vi "BuildStepListFromSteps.vi"(0 "Steps":T2(array[cluster]), 5 "Control Channels":string[](array[string]), 7 "Feedback Channels":string[](array[string]), 9 "AI":string[](array[string])) -> (4 "Step List":string[](array[string]))   [LabVIEW 2015]
panel:
  in  "Step":T1
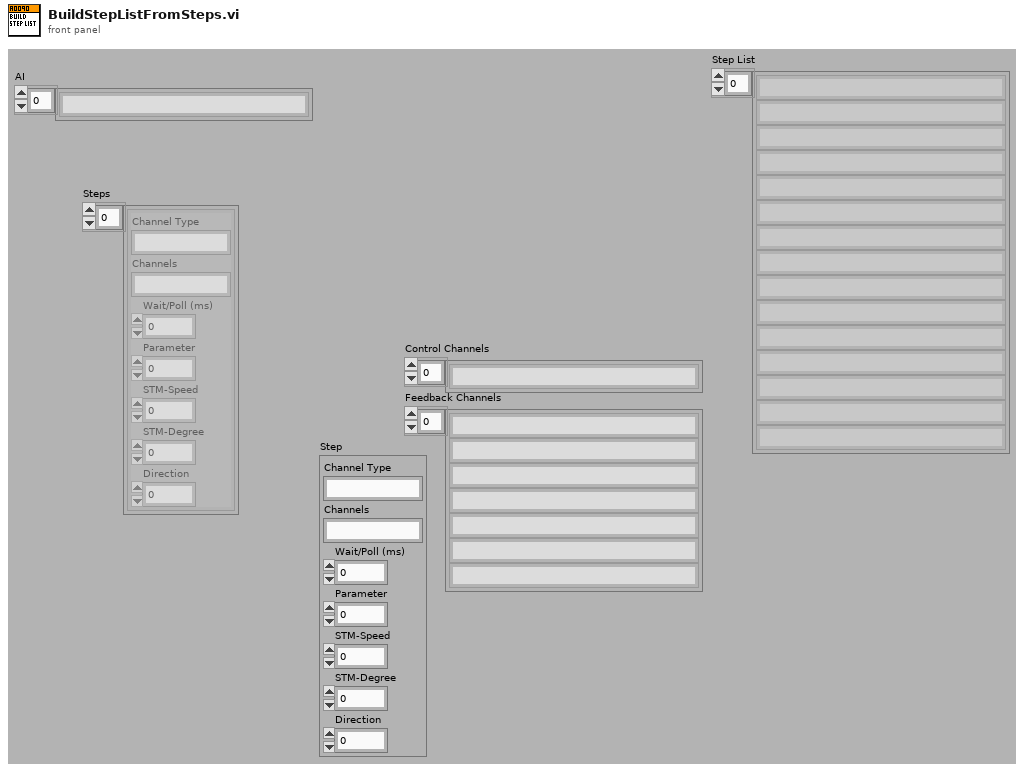
[diagram p1: front panel]
types:
  T1 = cluster{"Channel Type":string, "Channels":string, "Wait/Poll (ms)":u32, "Parameter":u8, "STM-Speed":u8, "STM-Degree":u32, "Direction":u8}
  T2 = cluster{"Channel Type":string, "Channels":string, "Wait/Poll (ms)":u32, "Parameter":u8, "STM-Speed":i32, "STM-Degree":u32, "Direction":u8}[]
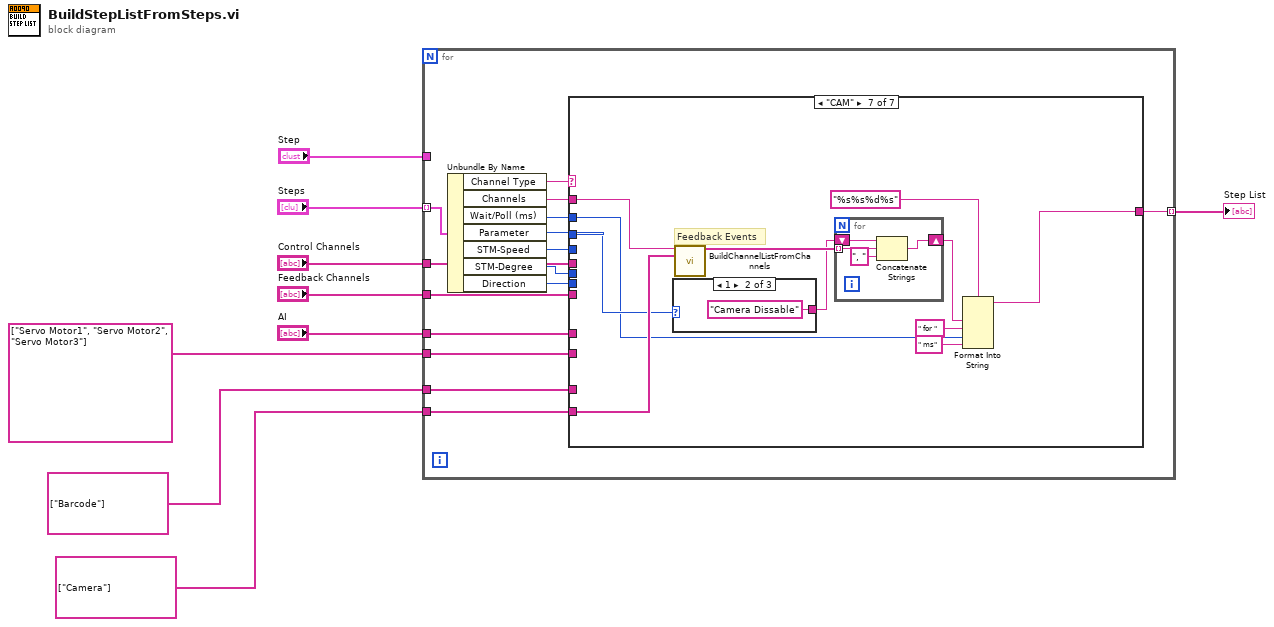
[diagram p0: block diagram]
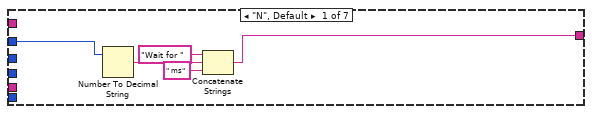
[diagram p2: hidden frame]
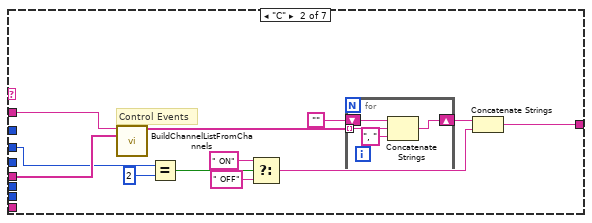
[diagram p3: hidden frame]
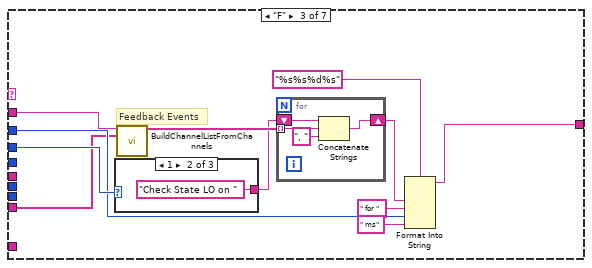
[diagram p4: hidden frame]
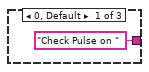
[diagram p5: hidden frame]
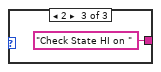
[diagram p6: hidden frame]
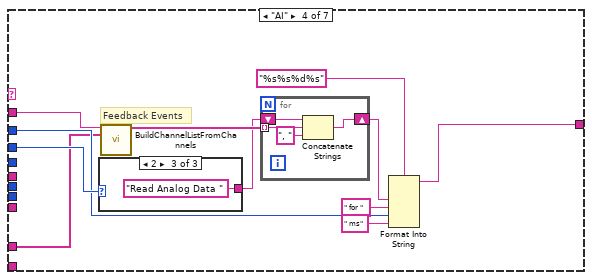
[diagram p7: hidden frame]
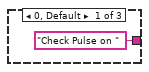
[diagram p8: hidden frame]
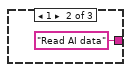
[diagram p9: hidden frame]
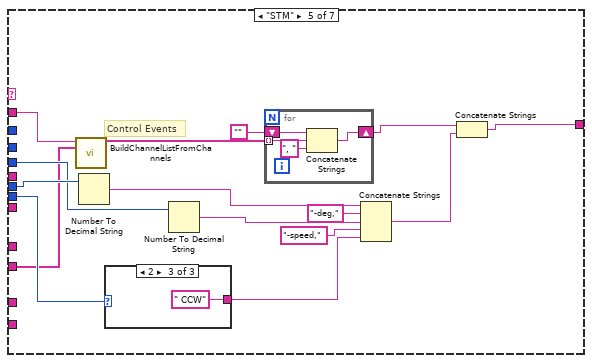
[diagram p10: hidden frame]
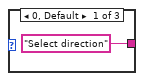
[diagram p11: hidden frame]
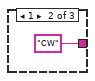
[diagram p12: hidden frame]
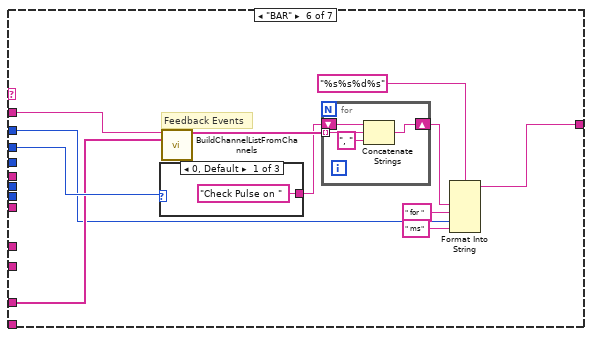
[diagram p13: hidden frame]
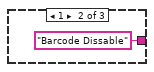
[diagram p14: hidden frame]
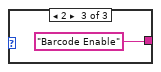
[diagram p15: hidden frame]
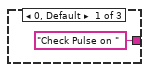
[diagram p16: hidden frame]
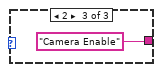
[diagram p17: hidden frame]
diagram:
  n1 = for {
    tunnel: "Steps" -> [w24] mode=indexing
    tunnel: "Control Channels" -> [w20]
    tunnel: "Feedback Channels" -> [w18]
    tunnel: [w17] -> w6 mode=indexing
    tunnel: "Step" -> [_]
    tunnel: "AI" -> [w16]
    tunnel: string[] ["Servo Motor1", "Servo Motor2", "Servo Motor3"] ("Control Channels 2") -> [w12]
    tunnel: string[] ["Barcode"] ("Channel Names (In)") -> [w11]
    tunnel: string[] ["Camera"] ("Channel Names (In)") -> [w10]
    n2 = Unbundle By Name(w24) -> ("Channel Type"=w23:string, "Channels"=w21:string, "Wait/Poll (ms)"=w22:u32, "Parameter"=w19:u8, "STM-Speed"=w13:i32, "STM-Degree"=w14:u32, "Direction"=w15:u8)
    n3 = case shown="\"CAM\"" w23 {
      tunnel: w22 -> [w26 _ w51 w67 _ w104 w123]
      tunnel: w21 -> [_ w41 w56 w66 w82 w107 w126]
      tunnel: w20 -> [_ w40 _ _ _ _ _]
      tunnel: w19 -> [_ w35 w52 w68 _ w108 w124]
      tunnel: w18 -> [_ _ w50 _ _ _ _]
      tunnel: [w25 w30 w47 w65 w92 w105 w122] -> w17
      tunnel: w16 -> [_ _ _ w64 _ _ _]
      tunnel: w15 -> [_ _ _ _ w93 _ _]
      tunnel: w14 -> [_ _ _ _ w91 _ _]
      tunnel: w13 -> [_ _ _ _ w88 _ _]
      tunnel: w12 -> [_ _ _ _ w83 _ _]
      tunnel: w11 -> [_ _ _ _ _ w106 _]
      tunnel: w10 -> [_ _ _ _ _ _ w125]
      frame "N", Default {
        n4 = Number To Decimal String(number=w26) -> (decimal integer string=w27:string)  [unwired: 1 in]
        n5 = Concatenate Strings("Wait for ", w27, " ms" ("string")) -> (w25:string)
      }
      frame "C" {
        # "Control Events"
        n6 = call "BuildChannelListFromChannels.vi"("Channels (A:B:C:D...) (In)"=w41, "Channel Names (In)"=w40) -> ("Channel List (Out)"=w34:string[])  [unwired: 12 in, 1 out]
        n7 = Equal?(x=w35, y=u8 2) -> (x = y?=w38:bool)
        n8 = Select(t=" ON", s=w38, f=" OFF") -> (s? t:f=w32:string)
        n9 = for {
          tunnel: w34 -> [w45] mode=indexing
          shift-right: [w42] -> w31
          shift-left: "" -> [w43]
          n10 = Concatenate Strings(w43, w45, ", " ("string")) -> (w42:string)
        }
        n11 = Concatenate Strings(w31, w32) -> (w30:string)
      }
      frame "F" {
        # "Feedback Events"
        n12 = case shown="1" w52 {
          tunnel: ["Check Pulse on " "Check State LO on " "Check State HI on "] -> w46
          frame 0, Default {
          }
          frame 1 {
          }
          frame 2 {
          }
        }
        n13 = call "BuildChannelListFromChannels.vi"("Channels (A:B:C:D...) (In)"=w56, "Channel Names (In)"=w50) -> ("Channel List (Out)"=w55:string[])  [unwired: 12 in, 1 out]
        n14 = for {
          tunnel: w55 -> [w63] mode=indexing
          shift-right: [w60] -> w48
          shift-left: w46 -> [w61]
          n15 = Concatenate Strings(w61, w63, ", " ("string")) -> (w60:string)
        }
        n16 = Format Into String(format string="%s%s%d%s", w48, " for " ("input 1"), w51, " ms" ("input 3")) -> (resulting string=w47:string)  [unwired: 2 in, 1 out]
      }
      frame "AI" {
        # "Feedback Events"
        n17 = case shown="2" w68 {
          tunnel: ["Check Pulse on " "Read AI data" "Read Analog Data "] -> w69
          frame 0, Default {
          }
          frame 1 {
          }
          frame 2 {
          }
        }
        n18 = call "BuildChannelListFromChannels.vi"("Channels (A:B:C:D...) (In)"=w66, "Channel Names (In)"=w64) -> ("Channel List (Out)"=w74:string[])  [unwired: 12 in, 1 out]
        n19 = for {
          tunnel: w74 -> [w81] mode=indexing
          shift-right: [w78] -> w70
          shift-left: w69 -> [w79]
          n20 = Concatenate Strings(w79, w81, ", " ("string")) -> (w78:string)
        }
        n21 = Format Into String(format string="%s%s%d%s", w70, " for " ("input 1"), w67, " ms" ("input 3")) -> (resulting string=w65:string)  [unwired: 2 in, 1 out]
      }
      frame "STM" {
        # "Control Events"
        n22 = call "BuildChannelListFromChannels.vi"("Channels (A:B:C:D...) (In)"=w82, "Channel Names (In)"=w83) -> ("Channel List (Out)"=w96:string[])  [unwired: 12 in, 1 out]
        n23 = Number To Decimal String(number=w91) -> (decimal integer string=w90:string)  [unwired: 1 in]
        n24 = case shown="2" w93 {
          tunnel: ["Select direction" "CW" " CCW"] -> w85
          frame 0, Default {
          }
          frame 1 {
          }
          frame 2 {
          }
        }
        n25 = Number To Decimal String(number=w88) -> (decimal integer string=w87:string)  [unwired: 1 in]
        n26 = for {
          tunnel: w96 -> [w103] mode=indexing
          shift-right: [w100] -> w94
          shift-left: "" -> [w101]
          n27 = Concatenate Strings(w101, w103, ", " ("string")) -> (w100:string)
        }
        n28 = Concatenate Strings(w90, "-deg," ("string"), w87, "-speed," ("string"), w85) -> (w84:string)
        n29 = Concatenate Strings(w94, w84) -> (w92:string)
      }
      frame "BAR" {
        # "Feedback Events"
        n30 = case shown="0, Default" w108 {
          tunnel: ["Check Pulse on " "Barcode Dissable" "Barcode Enable"] -> w109
          frame 0, Default {
          }
          frame 1 {
          }
          frame 2 {
          }
        }
        n31 = call "BuildChannelListFromChannels.vi"("Channels (A:B:C:D...) (In)"=w107, "Channel Names (In)"=w106) -> ("Channel List (Out)"=w114:string[])  [unwired: 12 in, 1 out]
        n32 = for {
          tunnel: w114 -> [w121] mode=indexing
          shift-right: [w118] -> w110
          shift-left: w109 -> [w119]
          n33 = Concatenate Strings(w119, w121, ", " ("string")) -> (w118:string)
        }
        n34 = Format Into String(format string="%s%s%d%s", w110, " for " ("input 1"), w104, " ms" ("input 3")) -> (resulting string=w105:string)  [unwired: 2 in, 1 out]
      }
      frame "CAM" {
        # "Feedback Events"
        n35 = case shown="1" w124 {
          tunnel: ["Check Pulse on " "Camera Dissable" "Camera Enable"] -> w127
          frame 0, Default {
          }
          frame 1 {
          }
          frame 2 {
          }
        }
        n36 = call "BuildChannelListFromChannels.vi"("Channels (A:B:C:D...) (In)"=w126, "Channel Names (In)"=w125) -> ("Channel List (Out)"=w132:string[])  [unwired: 12 in, 1 out]
        n37 = for {
          tunnel: w132 -> [w139] mode=indexing
          shift-right: [w136] -> w128
          shift-left: w127 -> [w137]
          n38 = Concatenate Strings(w137, w139, ", " ("string")) -> (w136:string)
        }
        n39 = Format Into String(format string="%s%s%d%s", w128, " for " ("input 1"), w123, " ms" ("input 3")) -> (resulting string=w122:string)  [unwired: 2 in, 1 out]
      }
    }
  }
  "Step List" <- w6
